vi "WT300 IEC 2015 Setup.vi"(0 "VISA Input":refnum<visa-resource-name>="WT210", 5 "Update Rate (250m s)":dbl(ring)=0.5 items=["100m"=0.1, "250m"=0.25, "500m"=0.5, "1"=1.0, "2"=2.0, "5"=5.0], 7 "Range Configuration (True)":bool[](array[boolean])=[FALSE, FALSE, FALSE, FALSE, FALSE, FALSE, FALSE, TRUE, TRUE, TRUE, TRUE, TRUE, FALSE], 11 "error in (no error)":errorcluster, 12 "Enable Auto Range (F: Disable)":bool=TRUE, 13 "Manual Range (20 <10> A)":dbl(ring)=10.0 items=["5m <2.5m>"=0.0025, "10m <5m>"=0.005, "20m <10m>"=0.01, "50m <25m>"=0.025, "100m <50m>"=0.05, "200m <100m>"=0.1, "500m <250m>"=0.25, "1 <500m>"=0.5, "2 <1>"=1.0, "5 <2.5>"=2.5, "10 <5>"=5.0, "20 <10>"=10.0, "40 <20>"=20.0]) -> (2 "VTHD":sgl=0.065 format="%.3g", 4 "VISA Output":refnum<visa-resource-name>="WT210", 6 "Header File":string[][](array[string])=[["Instrument", "YOKOGAWA,WT332,C2QB17128V,F1.03\n"], ["Instr Driver Revision", "1.0 F1.03"], ["Start Time", "1.0"], ["Voltage Range", "6/1/2015 11:50 AM"], ["Current Range", "Auto"], ["Update Rate", "Auto"], ["Standard", "0.250"], ["Algorithm", "IEC62301 Ed.2(Auto)"], ["Stop Factor", "Linear Regression"], ["Valid Period", ""], ["Start Total Harmonic Distortion Uthd 1", "0.065"], ["Start Total Harmonic Distortion Uthd 2", ""], ["End Total Harmonic Distortion Uthd 1", ""], ["End Total Harmonic Distortion Uthd 2", ""], ["Max Power (Watts)", ""], ["Power Variation (%)", ""], ["", ""]], 15 "error out":errorcluster)   [LabVIEW 2016]
uses:
  <vilib>/Utility/error.llb/whitespace.ctl
  Yokogawa WT300 Series.lvlib
  Public/Utility/Function/Create Function String (Harmonics).vi
  Public/Data/Read Measurement (Normal).vi
panel:
  out "Date & Time":string="6/1/2015 11:50 AM"
  out "Instrument ID":string="YOKOGAWA,WT332,C2QB17128V,F1.03\n"
  out "Sample Rate":string="0.250"
  # "5m <2.5m> A"
  # "10m <5m> A"
  # "20m <10m> A"
  # "50m <25m> A"
  # "100m <50m> A"
  # "200m <100m> A"
  # "500m <250m> A"
  # "1 <500m> A"
  # "2 <1> A"
  # "5 <2.5> A"
  # "10 <5> A"
  # "20 <10> A"
  # "40 <20> A"
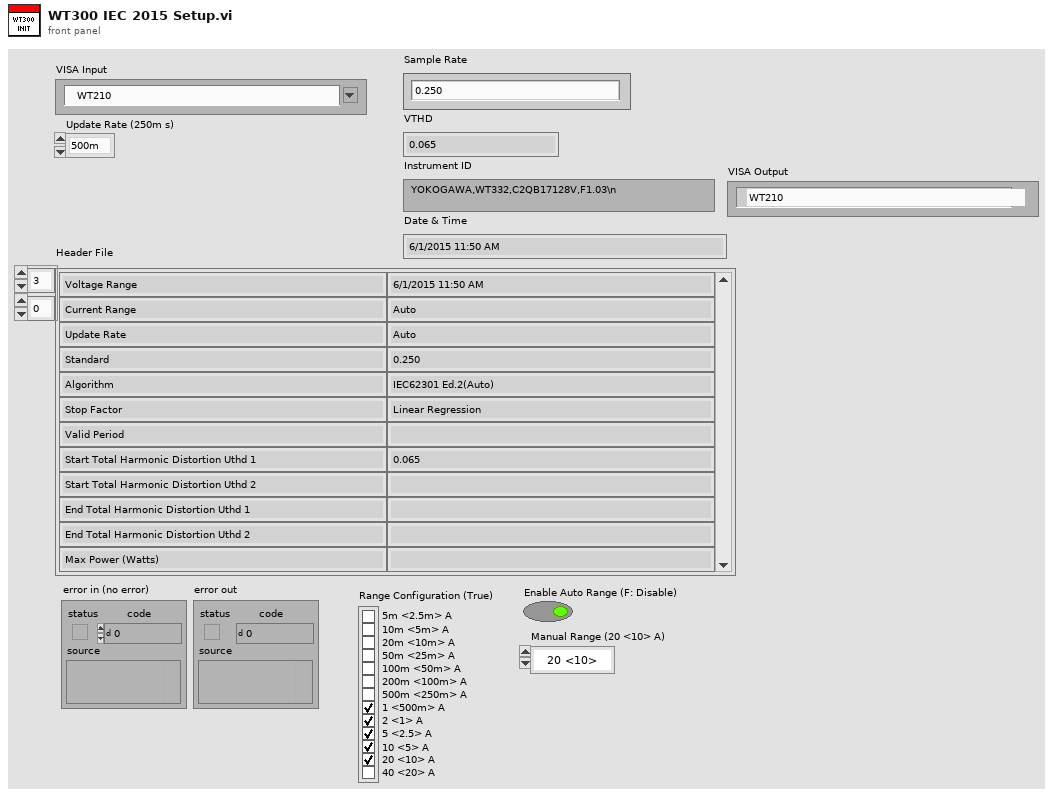
[diagram p1: front panel]
types:
  T1 = typedef "whitespace.ctl" = u16
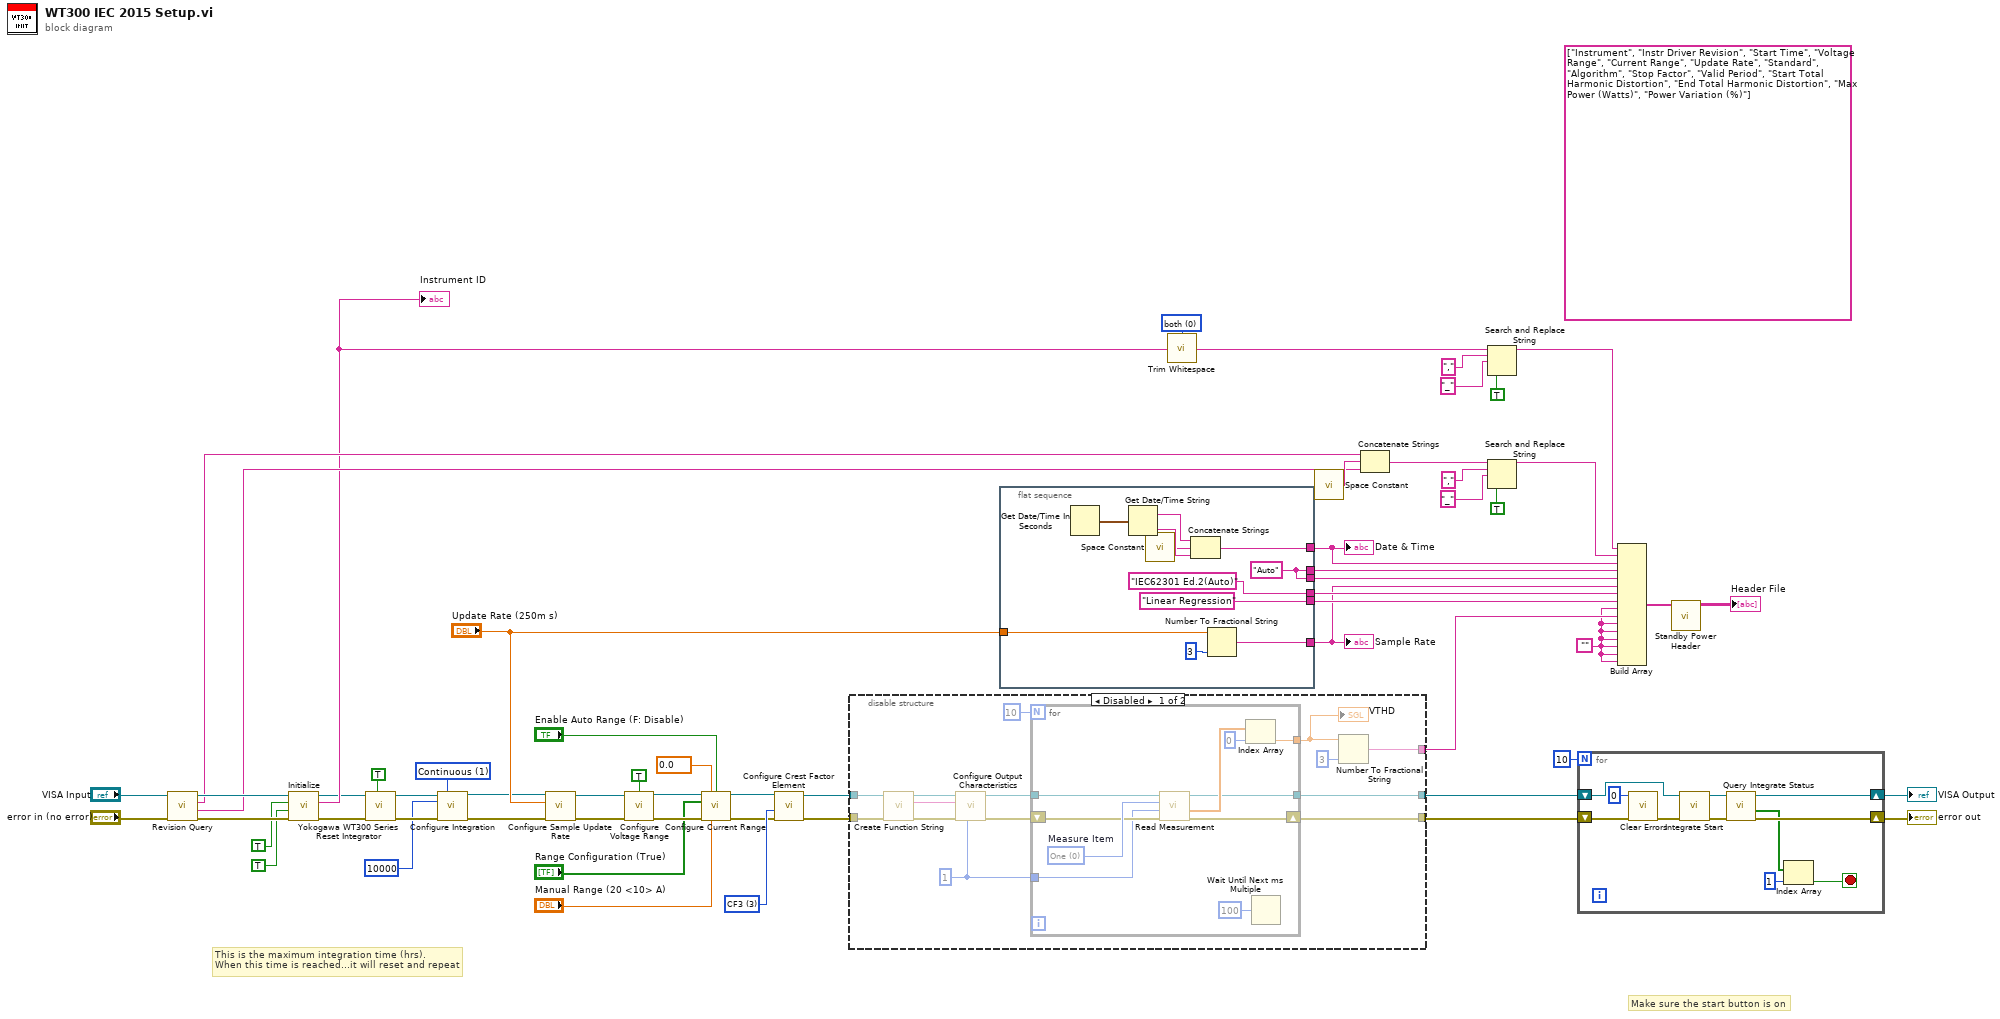
[diagram p0: block diagram]
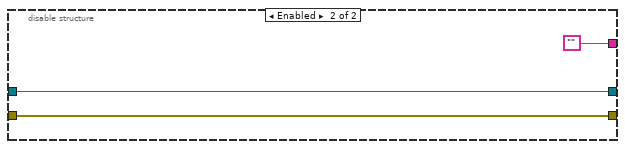
[diagram p2: hidden frame]
diagram:
  w1 = 0.0 items=["ALL", "Custom"] ("Range Type (1: Custom)")
  w7 = 1 items=["Normal", "Continuous"] ("Integration Mode (0: Normal)")
  w28 = T1 0 items=["both", "start of string", "end of string"] ("location (both)")
  w39 = 3 items=["CF3"=3, "CF6"=6] ("Crest Factor (3: CF3)")
  w34 = ""
  (unwired) string[] ["Instrument", "Instr Driver Revision", "Start Time", "Voltage Range", "Current Range", "Update Rate", "Standard", "Algorithm", "Stop Factor", "Valid Period", "Start Total Harmonic Distortion", "End Total Harmonic Distortion", "Max Power (Watts)", "Power Variation (%)"]
  # "Make sure the start button is on"
  # "This is the maximum integration time (hrs).\nWhen this time is reached...it will reset and repeat"
  n1 = call "Revision Query.vi"("error in (no error)"="error in (no error)", "VISA resource name"="VISA Input") -> ("error out"=w47:errorcluster, "Instrument Firmware Revision"=w48:string, "Instrument Driver Revision"=w49:string, "VISA resource name out"=w50:refnum<visa-resource-name>)  [unwired: 6 in]
  n2 = call "Initialize.vi"("error in (no error)"=w47, "Reset (True)"=TRUE, "ID Query (True)"=TRUE ("Reset (True)"), "VISA resource name"=w50) -> ("error out"=w12:errorcluster, "Instrument ID"=w29:string, "VISA resource name out"=w13:refnum<visa-resource-name>)  [unwired: 5 in]
  "Instrument ID" <- w29
  n3 = call "Yokogawa WT300 Series Reset Integrator.vi"("Initialization Routing?"=TRUE, "Error In"=w12, "VISA Refnum in"=w13) -> ("Error Out"=w11:errorcluster, "VISA resource name out"=w9:refnum<visa-resource-name>)  [unwired: 7 in]
  n4 = call "Configure Integration.vi"("VISA resource name"=w9, "Integration Mode (0: Normal)"=w7, "Integration Time Hour (0)"=10000, "error in (no error)"=w11) -> ("VISA resource name out"=w8:refnum<visa-resource-name>, "error out"=w10:errorcluster)  [unwired: 10 in]
  n5 = call "Configure Sample Update Rate.vi"("error in (no error)"=w10, "Update Rate (500m s)"="Update Rate (250m s)", "VISA resource name"=w8) -> ("error out"=w46:errorcluster, "VISA resource name out"=w44:refnum<visa-resource-name>)  [unwired: 7 in]
  n6 = call "Configure Voltage Range.vi"("VISA resource name"=w44, "Enable Auto Range (F: Disable)"=TRUE, "error in (no error)"=w46) -> ("VISA resource name out"=w43:refnum<visa-resource-name>, "error out"=w42:errorcluster)  [unwired: 11 in]
  n7 = call "Configure Current Range.vi"("VISA resource name"=w43, "Range Type (1: Custom)"=w1, "Enable Auto Range (F: Disable)"="Enable Auto Range (F: Disable)", "Range Configuration (True)"="Range Configuration (True)", "error in (no error)"=w42, "Manual Range (20 <10> A)"="Manual Range (20 <10> A)") -> ("VISA resource name out"=w37:refnum<visa-resource-name>, "error out"=w38:errorcluster)  [unwired: 8 in]
  n8 = call "Configure Crest Factor Element.vi"("error in (no error)"=w38, "Crest Factor (3: CF3)"=w39, "VISA resource name"=w37) -> ("error out"=w33:errorcluster, "VISA resource name out"=w32:refnum<visa-resource-name>)  [unwired: 7 in]
  n9 = disable-structure shown="Disabled" {
    disable-tunnel: [w71 ""] -> w35
    disable-tunnel: w33 -> [w67 w87]
    disable-tunnel: w32 -> [w66 w86]
    disable-tunnel: [w62 w87] -> w31
    disable-tunnel: [w61 w86] -> w30
    frame Disabled {
      w63 = 1 ("Item (1)")
      n10 = call-poly "Create Function String.vi"("error in (no error)"=w67, "VISA resource name"=w66) -> ("error out"=w68:errorcluster, "Function String"=w69:string, "VISA resource name out"=w70:refnum<visa-resource-name>)  [unwired: 7 in]
      n11 = call "Configure Output Characteristics.vi"("Item (1)"=w63, "error in (no error)"=w68, "Function (Empty)"=w69, "VISA resource name"=w70) -> ("error out"=w64:errorcluster, "VISA resource name out"=w65:refnum<visa-resource-name>)  [unwired: 6 in]
      n12 = for {
        N: 10 -> [_]
        tunnel: w65 -> [w81]
        tunnel: w63 -> [w79]
        tunnel: [w77] -> w61
        tunnel: [w76] -> w73
        shift-right: [w78] -> w62
        shift-left: w64 -> [w80]
        w82 = 0 items=["One", "Plural"]  # Measure Item
        n13 = call-poly "Read Measurement.vi"("error in (no error)"=w80, "Number of Item (15)"=w79, "Measure Item (1: Plural)"=w82, "VISA resource name"=w81) -> ("error out"=w78:errorcluster, "Measurement"=w83:dbl[], "VISA resource name out"=w77:refnum<visa-resource-name>)  [unwired: 4 in, 1 out]
        n14 = Index Array(array=w83, index=0 ("指標 （行）")) -> (element=w76:dbl)
        n15 = Wait Until Next ms Multiple(millisecond multiple=u32 100) -> ()  [unwired: 1 out]
      }
      "VTHD" <- w73
      n16 = Number To Fractional String(number=w73, precision (6)=i16 3) -> (F-format string=w71:string)  [unwired: 2 in]
    }
    frame Enabled {
    }
  }
  n17 = flat-sequence {
    tunnel: [w91] -> w60
    tunnel: [w91] -> w59
    tunnel: ["IEC62301 Ed.2(Auto)" ("element")] -> w58
    tunnel: ["Linear Regression" ("element")] -> w57
    tunnel: [w92] -> w54
    tunnel: [w90] -> w53
    tunnel: "Update Rate (250m s)" -> [w89]
    frame #0 {
      w91 = "Auto"
      n18 = Get Date/Time In Seconds() -> (seconds since 1Jan1904=w93:timestamp)
      n19 = Get Date/Time String(seconds (now)=w93) -> (date string=w95:string, time string=w96:string)  [unwired: 2 in]
      n20 = call <vilib>:"Space Constant.vi"() -> ("String"=w94:string)
      n21 = Concatenate Strings(w95, w94, w96) -> (w92:string)
      n22 = Number To Fractional String(number=w89, precision (6)=i16 3) -> (F-format string=w90:string)  [unwired: 2 in]
    }
  }
  n23 = call <vilib>:"Trim Whitespace.vi"("string"=w29, "location (both)"=w28) -> ("trimmed string"=w18:string)
  n24 = call <vilib>:"Space Constant.vi"() -> ("String"=w55:string)
  n25 = Concatenate Strings(w49, w55, w48) -> (w23:string)
  n26 = Search and Replace String(replace all?=TRUE ("replace all? (F)"), input string=w18, search string=",", replace string="_" ("replace string (\"\")")) -> (result string=w17:string)  [unwired: 4 in, 3 out]
  n27 = Search and Replace String(replace all?=TRUE ("replace all? (F)"), input string=w23, search string=",", replace string="_" ("replace string (\"\")")) -> (result string=w22:string)  [unwired: 4 in, 3 out]
  n28 = for {
    N: 10 -> [_]
    shift-right: [w105] -> w4
    shift-left: w31 -> [w101]
    shift-right: [w106] -> w5
    shift-left: w30 -> [w109]
    stop <- w102 stop-if-true
    n29 = call <vilib>:"Clear Errors.vi"("error in (no error)"=w101, "specific error code to clear (0: all)"=0) -> ("error out"=w100:errorcluster)  [unwired: 4 in, 1 out]
    n30 = call "Integrate Start.vi"("error in (no error)"=w100, "VISA resource name"=w109) -> ("error out"=w107:errorcluster, "VISA resource name out"=w108:refnum<visa-resource-name>)  [unwired: 8 in]
    n31 = call "Query Integrate Status.vi"("error in (no error)"=w107, "VISA resource name"=w108) -> ("error out"=w105:errorcluster, "Integrate Status List"=w104:bool[], "VISA resource name out"=w106:refnum<visa-resource-name>)  [unwired: 6 in, 1 out]
    n32 = Index Array(array=w104, index=1) -> (element=w102:bool)
  }
  "error out" <- w4
  "VISA Output" <- w5
  n33 = Build Array(w17, w22, w54, w60, w59, w53, w58, w57, w34, w35, w34, w34, w34, w34, w34, w34) -> (w56:string[])
  n34 = call "Standby Power Header.vi"("Array"=w56) -> ("Header File"=→"Header File":string[][])  [unwired: 9 in, 1 out]
  "Sample Rate" <- w53
  "Date & Time" <- w54
